vi "Main.vi"(11 "_Rescript Msg in":refnum<class "_Rescript Msg.lvclass">) -> ()   [LabVIEW 2021, in "_Rescript Msg.lvlib" / "_Rescript Msg.lvclass"]
uses:
  _Rescript Msg.lvclass
  _Rescript Msg.lvclass/_Rescript Msg.ctl
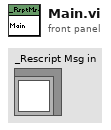
[diagram p1: front panel]
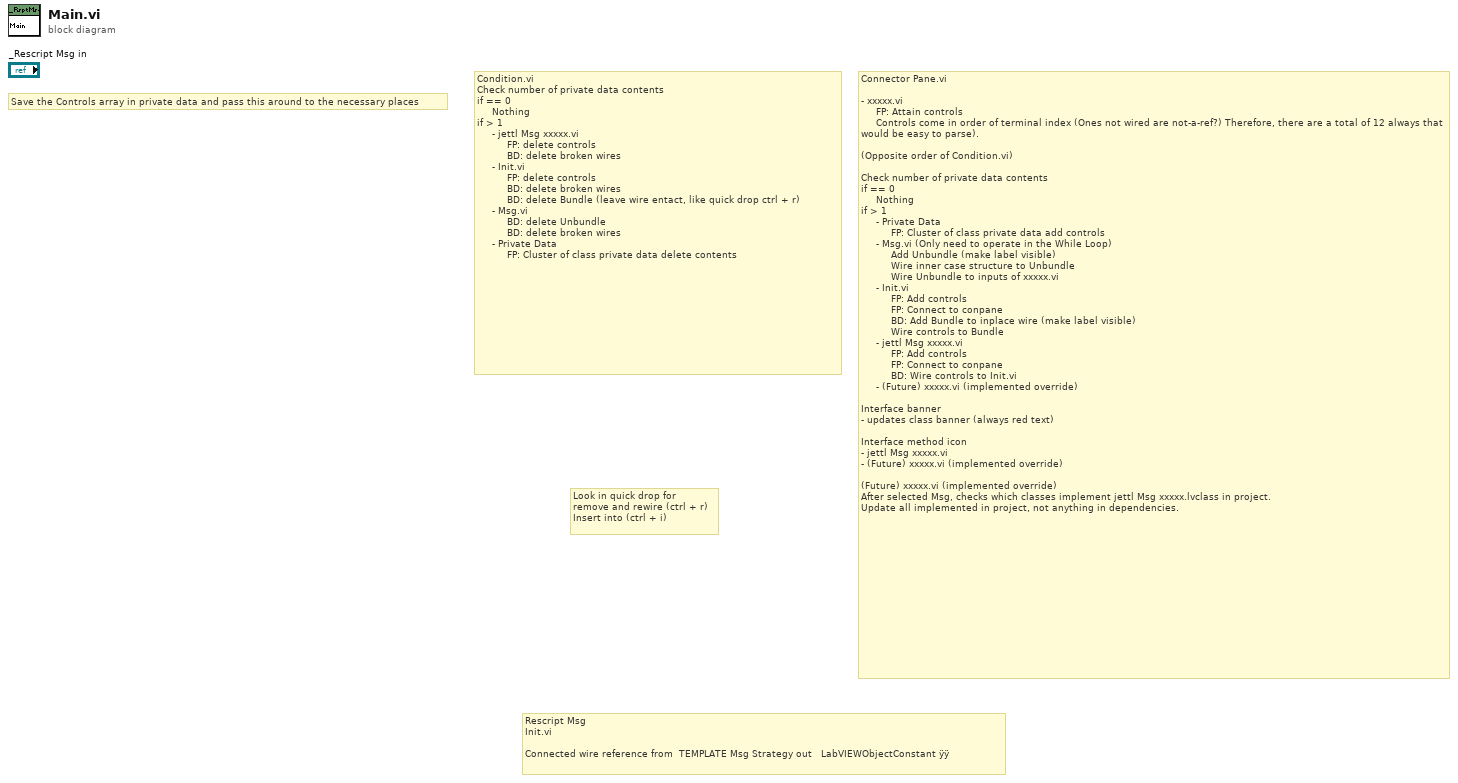
[diagram p0: block diagram]
diagram:
  # "Rescript Msg\nInit.vi\n\nConnected wire reference from  TEMPLATE Msg Strategy out   LabVIEWObjectConstant ÿÿ"
  # "Look in quick drop for\nremove and rewire (ctrl + r)\nInsert into (ctrl + i)"
  # "Connector Pane.vi\n\n- xxxxx.vi\n     FP: Attain controls\n     Controls come in order of terminal index (Ones not wired are not-a-ref?) Therefore, there are a total of 12 always that would be easy to parse).\n\n(Opposite order of Condition.vi)\n\nCheck number of private data contents\nif == 0\n     Nothing\nif > 1\n     - Private Data\n          FP: Cluster of class private data add controls\n     - Msg.vi (Only need to operate in the While Loop)\n          Add Unbundle (make label visible)\n          Wire inner case structure to Unbundle\n          Wire Unbundle to inputs of xxxxx.vi\n     - Init.vi\n          FP: Add controls\n          FP: Connect to conpane\n          BD: Add Bundle to inplace wire (make label visible)\n          Wire controls to Bundle\n     - jettl Msg xxxxx.vi\n          FP: Add controls\n          FP: Connect to conpane\n          BD: Wire controls to Init.vi\n     - (Future) xxxxx.vi (implemented override)\n\nInterface banner\n- updates class banner (always red text)\n\nInterface method icon\n- jettl Msg xxxxx.vi\n- (Future) xxxxx.vi (implemented override)\n\n(Future) xxxxx.vi (implemented override)\nAfter selected Msg, checks which classes implement jettl Msg xxxxx.lvclass in project.\nUpdate all implemented in project, not anything in dependencies."
  # "Condition.vi\nCheck number of private data contents\nif == 0\n     Nothing\nif > 1\n     - jettl Msg xxxxx.vi\n          FP: delete controls\n          BD: delete broken wires\n     - Init.vi\n          FP: delete controls\n          BD: delete broken wires\n          BD: delete Bundle (leave wire entact, like quick drop ctrl + r)\n     - Msg.vi\n          BD: delete Unbundle\n          BD: delete broken wires\n     - Private Data\n          FP: Cluster of class private data delete contents"
  # "Save the Controls array in private data and pass this around to the necessary places"
